vi "Main.vi"() -> (0 "Image Out":T1(plugin-control))   [LabVIEW 2013]
uses:
  <vilib>/ptbypt/NI_PtbyPt.lvlib
panel:
  in  "Manual Value Set":bool
  in  "Brightness":i32=128
  in  "Exposure":i32=4000
  out "Brightness":i32
  out "Exposure":i32
  out "Input Voltage":dbl
  out "Obstacle Case":u8
  in  "Avoid Distance":dbl=0.75 format="%#_13g"
  out "Roll":dbl
  out "Pitch":dbl
  out "Case":i32
  in  "Negative (Reverse) \nPitch Limit":dbl=-0.2
  in  "Positive (Forward) \nPitch Limit":dbl=0.6
  in  "Roll Limit":dbl=0.4
  out "Right":dbl
  out "Left":dbl
  out "Obstacle Detected":bool
  in  "Color Mode":u16(ring) items=["RGB", "HSL", "HSV", "HSI"]
  in  "Red Range":cluster{"Lower value":i32, "Upper value":i32}={"Lower value"=200, "Upper value"=255}
  in  "Green Range":cluster{"Lower value":i32, "Upper value":i32}={"Lower value"=200, "Upper value"=255}
  in  "Blue Range":cluster{"Lower value":i32, "Upper value":i32}={"Lower value"=200, "Upper value"=230}
  in  "Centroid \n  Offset":dbl=15.0
  out "Center X":dbl
  out "Center Y":sgl
  out "Vision Case":i32
  in  "Centroid\nSamples":i32=3
  in  "US Average\nLength":i32=5
  in  "Motor Enable":bool
  in  "Sunlight Brightness":i64=100
  in  "Sunlight Exposure":i64=10000
  in  "Shade Brightness":i64=128
  in  "Shade Exposure":i64=2000
  out "Frame Rate":dbl
  in  "Steering":dbl(slide) caption="Servo Control" step=10.0 scale=-100.0..100.0
  in  "Speed":dbl(knob) step=10.0 scale=-100.0..100.0
  in  "STOP":bool
  in  "Motor \nFrequency":dbl=2500.0
  in  "Manual/Autonomous":bool
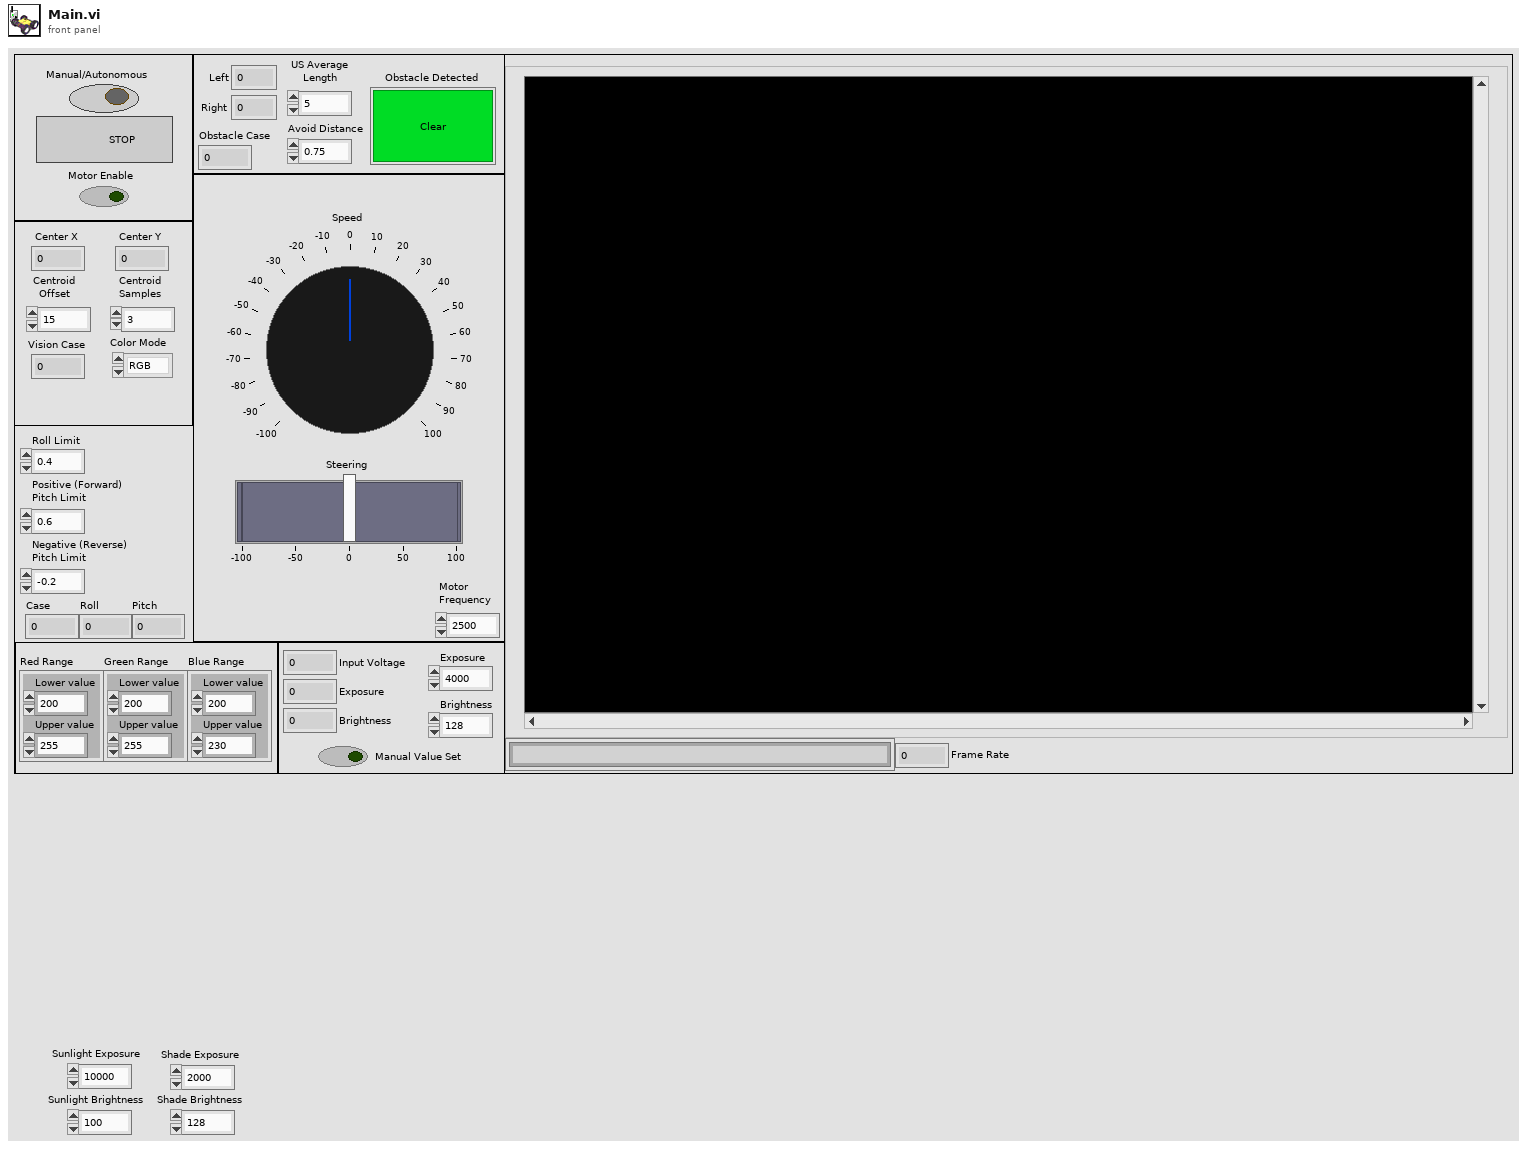
[diagram p1: front panel]
types:
  T1 = typedef "IMAQ Image.ctl" = refnum<image>
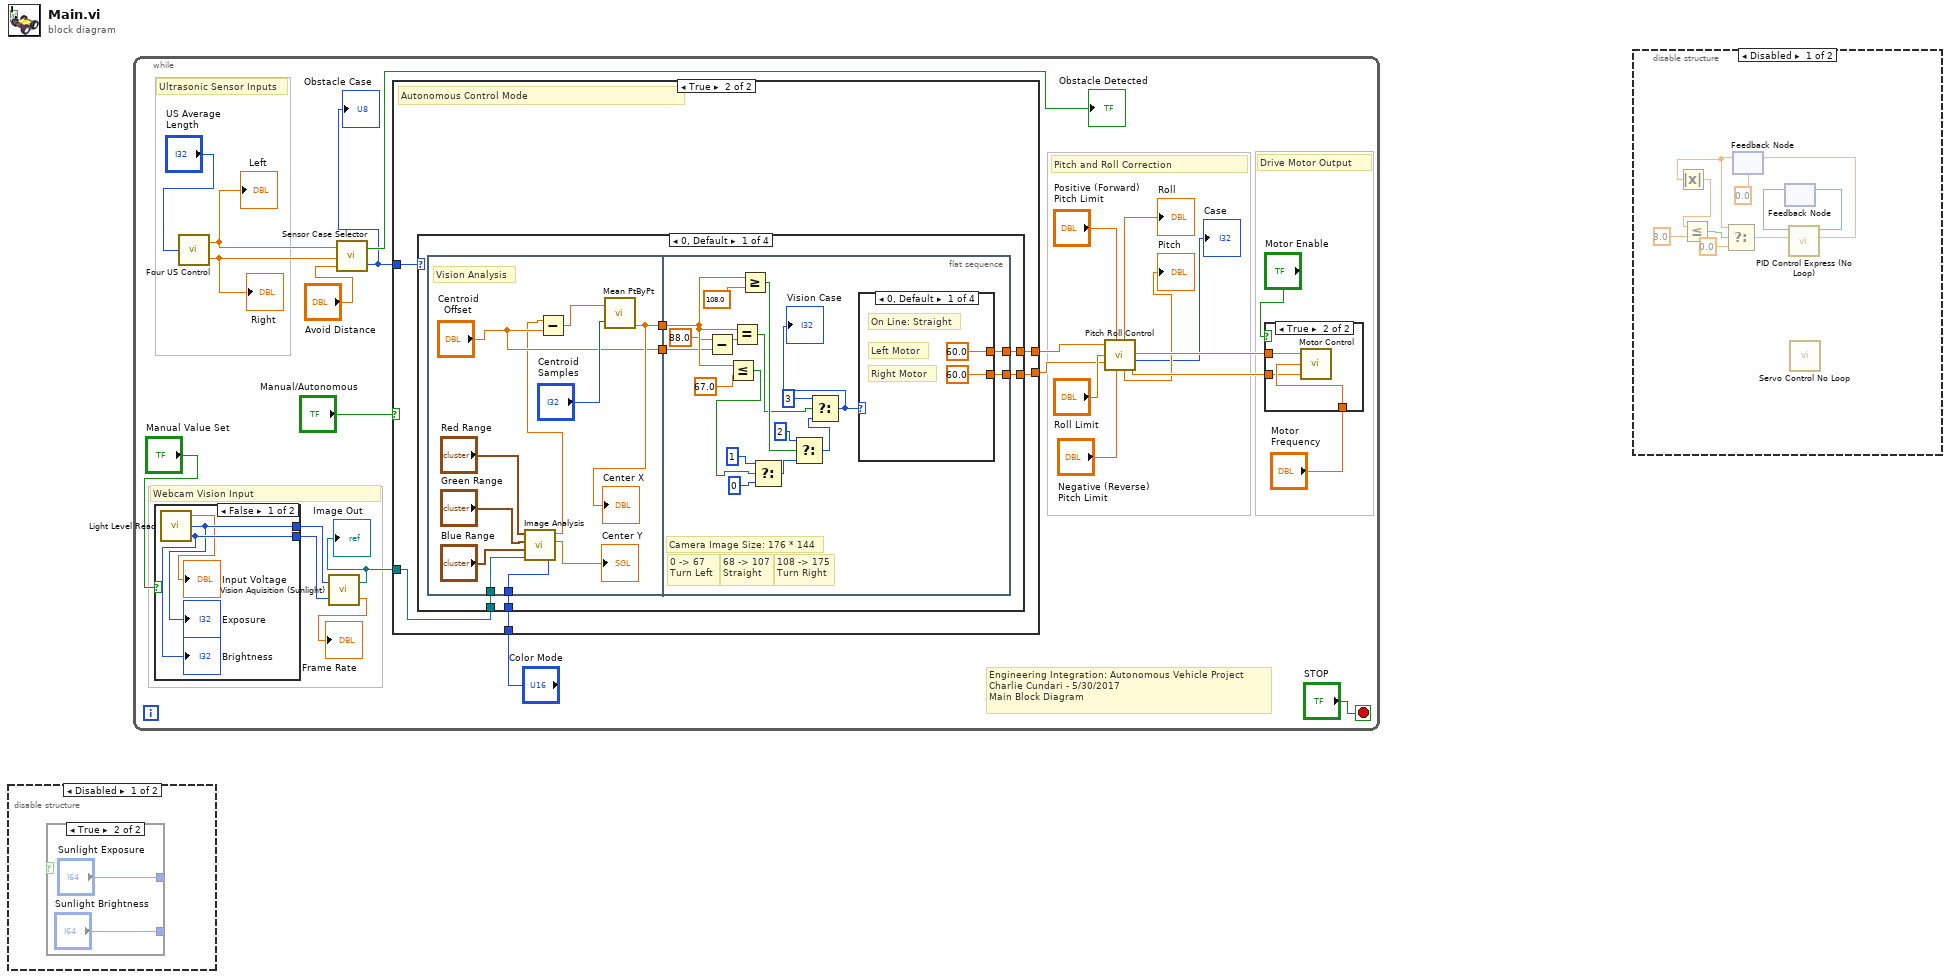
[diagram p0: block diagram]
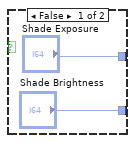
[diagram p2: hidden frame]
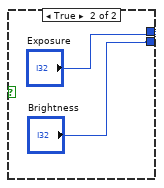
[diagram p5: hidden frame]
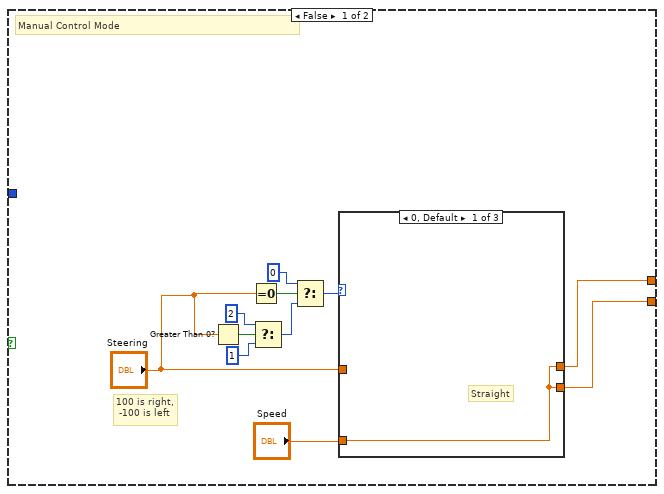
[diagram p7: hidden frame]
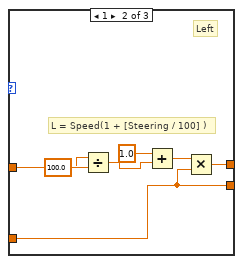
[diagram p8: hidden frame]
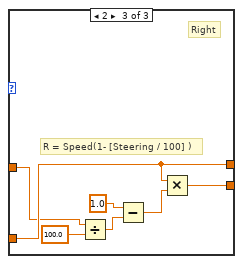
[diagram p9: hidden frame]
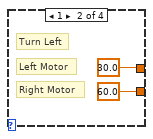
[diagram p10: hidden frame]
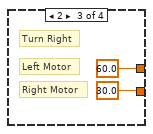
[diagram p11: hidden frame]
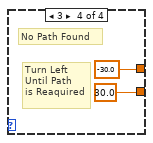
[diagram p12: hidden frame]
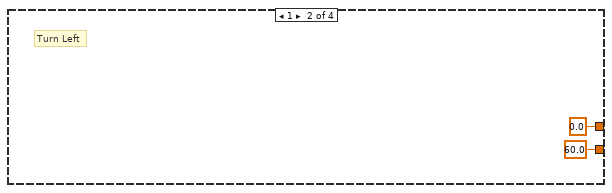
[diagram p13: hidden frame]
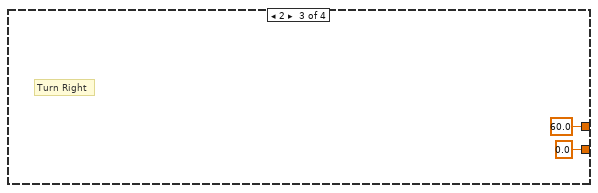
[diagram p14: hidden frame]
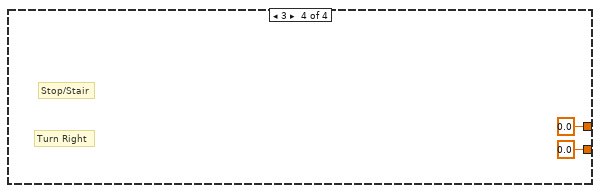
[diagram p15: hidden frame]
diagram:
  n1 = disable-structure shown="Disabled" {
    frame Disabled {
      n2 = case shown="True" {
        selector: _ -> [_ _]
        tunnel: ["Shade Exposure" "Sunlight Exposure"] -> _
        tunnel: ["Shade Brightness" "Sunlight Brightness"] -> _
        frame False {
        }
        frame True {
        }
      }
    }
    frame Enabled {
    }
  }
  n3 = while {
    stop <- "STOP" stop-if-true
    # "Engineering Integration: Autonomous Vehicle Project\nCharlie Cundari - 5/30/2017\nMain Block Diagram"
    # "Ultrasonic Sensor Inputs"
    # "Pitch and Roll Correction"
    # "Drive Motor Output"
    # "Webcam Vision Input"
    n4 = case shown="False" "Manual Value Set" {
      tunnel: [w33 "Brightness"] -> w12
      tunnel: [w32 "Exposure"] -> w11
      frame False {
        n5 = call "Light Level Read.vi"() -> ("Brightness"=w33:i32, "Exposure"=w32:i32, "Input Voltage (A3)"=→"Input Voltage":dbl)
        "Exposure" <- w32
        "Brightness" <- w33
      }
      frame True {
      }
    }
    n6 = call "Four US Control.vi"("Average Length"="US Average\nLength") -> ("Distance Front\nRight (A11)"=w22:dbl, "Distance Front\nLeft (A13)"=w23:dbl)  [unwired: 2 out]
    "Left" <- w23
    "Right" <- w22
    n7 = call "Vision Aquisition (Sunlight).vi"("Brightness::Value"=w12, "Exposure::Value"=w11) -> ("Frame Rate"=→"Frame Rate":dbl, "Image Out"=w5:T1)
    "Image Out" <- w5
    n8 = call "Sensor Case Selector.vi"("Avoid Distance"="Avoid Distance", "FR"=w22, "FL"=w23) -> ("Case"=w13:u8, "Obstacle Detected"=→"Obstacle Detected":bool)
    "Obstacle Case" <- w13
    n9 = case shown="True" "Manual/Autonomous" {
      tunnel: [w42 w68] -> w9
      tunnel: [w41 w69] -> w15
      tunnel: "Color Mode" -> [_ w67]
      tunnel: w13 -> [_ w66]
      tunnel: w5 -> [_ w65]
      frame False {
        # "100 is right,\n -100 is left"
        # "Manual Control Mode"
        n10 = Greater Than 0?(x="Steering") -> (x > 0?=w46:bool)
        n11 = Equal To 0?(x="Steering") -> (x = 0?=w49:bool)
        n12 = Select(t=2, s=w46, f=1 ("t")) -> (s? t:f=w45:i32)
        n13 = Select(t=0, s=w49, f=w45) -> (s? t:f=w47:i32)
        n14 = case shown="0, Default" w47 {
          tunnel: "Speed" -> [w50 w53 w59]
          tunnel: [w50 w53 w64] -> w42
          tunnel: [w50 w54 w59] -> w41
          tunnel: "Steering" -> [_ w55 w58]
          frame 0, Default {
            # "Straight"
          }
          frame 1 {
            # "L = Speed(1 + [Steering / 100] )"
            # "Left"
            n15 = Divide(x=w55, y=100.0) -> (x/y=w51:dbl)
            n16 = Add(x=1.0, y=w51) -> (x+y=w52:dbl)
            n17 = Multiply(x=w52, y=w53) -> (x*y=w54:dbl)
          }
          frame 2 {
            # "R = Speed(1- [Steering / 100] )"
            # "Right"
            n18 = Divide(x=w58, y=100.0) -> (x/y=w61:dbl)
            n19 = Subtract(x=1.0, y=w61) -> (x-y=w60:dbl)
            n20 = Multiply(x=w59, y=w60) -> (x*y=w64:dbl)
          }
        }
      }
      frame True {
        # "Autonomous Control Mode"
        n21 = case shown="0, Default" w66 {
          tunnel: [w74 0.0 60.0 0.0] -> w69
          tunnel: [w73 60.0 0.0 0.0] -> w68
          tunnel: w67 -> [w72 _ _ _]
          tunnel: w65 -> [w70 _ _ _]
          frame 0, Default {
            n22 = flat-sequence {
              tunnel: [w80] -> w75
              tunnel: w72 -> [w81]
              tunnel: ["Centroid \n  Offset"] -> w71
              tunnel: w70 -> [w76]
              tunnel: w75 -> [w89]
              tunnel: [w99] -> w73
              tunnel: [w98] -> w74
              tunnel: w71 -> [w88]
              frame #0 {
                # "Vision Analysis"
                n23 = call "Image Analysis.vi"("Color Mode (Color Threshold 1)"=w81, "Image In"=w76, "Blue or Luma or Val or Inten Range"="Blue Range", "Green or Sat Range"="Green Range", "Red or Hue Range"="Red Range") -> ("Y Centroid"=→"Center Y":sgl, "X Centroid"=w78:sgl)  [unwired: 1 out]
                n24 = Subtract(x=w78, y="Centroid \n  Offset") -> (x-y=w86:dbl)
                n25 = call <vilib>:"Mean PtByPt.vi"("x"=w86, "sample length"="Centroid\nSamples") -> ("mean"=w80:dbl)  [unwired: 2 in, 1 out]
                "Center X" <- w80
              }
              frame #1 {
                # "68 -> 107\nStraight"
                # "108 -> 175\nTurn Right"
                # "0 -> 67\nTurn Left"
                # "Camera Image Size: 176 * 144"
                n26 = Subtract(x=88.0, y=w88) -> (x-y=w90:dbl)
                n27 = Less Or Equal?(x=w89, y=67.0) -> (x <= y?=w97:bool)
                n28 = Equal?(x=w89, y=w90) -> (x = y?=w92:bool)
                n29 = Greater Or Equal?(x=w89, y=108.0) -> (x >= y?=w95:bool)
                n30 = Select(t=1, s=w97, f=0) -> (s? t:f=w104:i32)
                n31 = Select(t=2, s=w95, f=w104) -> (s? t:f=w93:i32)
                n32 = Select(t=3, s=w92, f=w93) -> (s? t:f=w94:i32)
                "Vision Case" <- w94
                n33 = case shown="0, Default" w94 {
                  tunnel: [60.0 60.0 30.0 30.0] -> w99
                  tunnel: [60.0 30.0 60.0 -30.0] -> w98
                  frame 0, Default {
                    # "Left Motor"
                    # "Right Motor"
                    # "On Line: Straight"
                  }
                  frame 1 {
                    # "Left Motor"
                    # "Right Motor"
                    # "Turn Left"
                  }
                  frame 2 {
                    # "Left Motor"
                    # "Right Motor"
                    # "Turn Right"
                  }
                  frame 3 {
                    # "Turn Left\nUntil Path\nis Reaquired"
                    # "No Path Found"
                  }
                }
              }
            }
          }
          frame 1 {
            # "Turn Left"
          }
          frame 2 {
            # "Turn Right"
          }
          frame 3 {
            # "Turn Right"
            # "Stop/Stair"
          }
        }
      }
    }
    n34 = call "Pitch Roll Control.vi"("Left Motor In"=w15, "Positive (Reverse) \nPitch Limit"="Positive (Forward) \nPitch Limit", "Roll Limit"="Roll Limit", "Right Motor In"=w9, "Negative (Forward) \nPitch Limit"="Negative (Reverse) \nPitch Limit") -> ("Roll"=→"Roll":dbl, "Left Motor Out"=w20:dbl, "Case"=→"Case":i32, "Pitch"=→"Pitch":dbl, "Right Motor Out"=w19:dbl)
    n35 = case shown="True" "Motor Enable" {
      tunnel: "Motor \nFrequency" -> [_ w38]
      tunnel: w20 -> [_ w37]
      tunnel: w19 -> [_ w36]
      frame False {
      }
      frame True {
        n36 = call "Motor Control.vi"("Right Motor"=w36, "Motor Frequency"=w38, "Left Motor"=w37) -> ()
      }
    }
  }
  n37 = disable-structure shown="Disabled" {
    frame Disabled {
      n38 = feedback #1(0.0 ("Control Out")) -> (w126:dbl)
      n39 = Absolute Value(x=w126) -> (abs(x)=w128:dbl)
      n40 = Less Or Equal?(x=w128, y=3.0) -> (x <= y?=w127:bool)
      n41 = Select(t=w126, s=w127, f=0.0) -> (s? t:f=w122:dbl)
      n42 = feedback #2() -> (w121:i32)  [unwired: 1 in]
      n43 = call "PID Control Express (No Loop).vi"("Control In"=w122, "Counter In"=w121) -> ("RPM Difference"=w133:dbl, "Mean RPM"=w132:dbl, "Control Out"=w123:dbl, "Counter Out"=w120:i32, "Kp"=w130:dbl, "DC Motor Frequency"=w131:dbl, "Motor Enable"=w134:bool)  [unwired: 1 in]
      n44 = feedback-in #1(w123) -> ()
      n45 = feedback-in #2(w120) -> ()
      n46 = call "Servo Control No Loop.vi"() -> ("Servo Angle"=w119:dbl)  [unwired: 1 in]
    }
    frame Enabled {
    }
  }
